vi "TimeInterpRotation_GetSample.vi"(9 "TimeStamp":dbl, 11 "TimeInterpRotation":T1 {"RotationValues"."SIN" format="%13.4f"; "RotationValues"."COS" format="%13.4f"; "RotationValues"."VALUE" format="%13.4f"}) -> (3 "OutputRotation":T2={"VALUE"=0.0, "COS"=1.0, "SIN"=0.0} {"SIN" format="%13.4f"; "COS" format="%13.4f"; "VALUE" format="%13.4f"})   [LabVIEW 2019, in "Trajectory_Library.lvlib"]
doc: "Calculate the output Y value for the provided X. This is done by interpolating through an array of X and Y pairs. The pairs must be ordered in increasing X value.\n\nInputs:\n - Function_Generator -- function generator data structure\n - Input Value -- The input value. \n\nOutputs:\n - Output Value -- Output value calcuated from the input value."
uses:
  Trajectory_Library.lvlib
  <vilib>/gmath/NI_Gmath.lvlib
  ROTATION2D.ctl
  TIME_INTERPOLATABLE_ROTATION.ctl
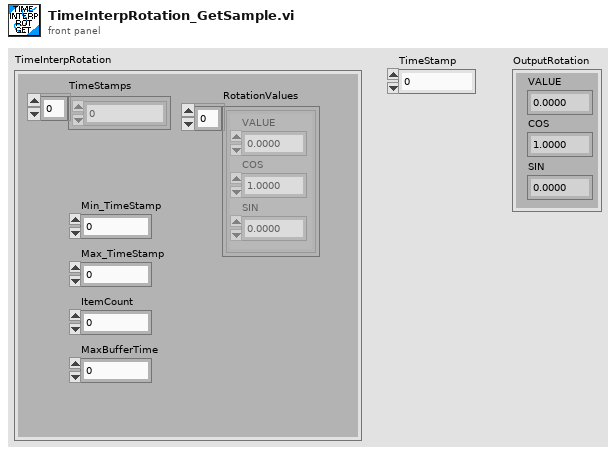
[diagram p1: front panel]
types:
  T1 = typedef "Trajectory_Library.lvlib/TIME_INTERPOLATABLE_ROTATION.ctl" = cluster{"TimeStamps":dbl[], "RotationValues":T2[], "Min_TimeStamp":dbl, "Max_TimeStamp":dbl, "ItemCount":i32, "MaxBufferTime":dbl}
  T2 = typedef "Trajectory_Library.lvlib/ROTATION2D.ctl" = cluster{"VALUE":dbl, "COS":dbl, "SIN":dbl}
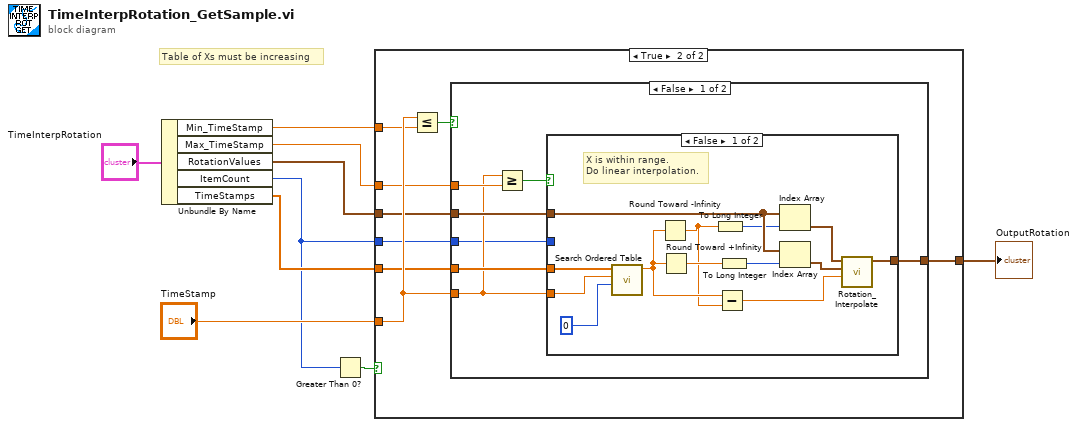
[diagram p0: block diagram]
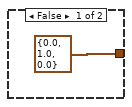
[diagram p2: hidden frame]
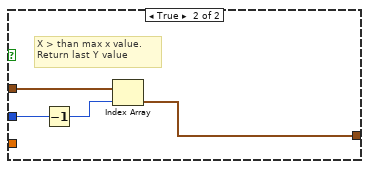
[diagram p3: hidden frame]
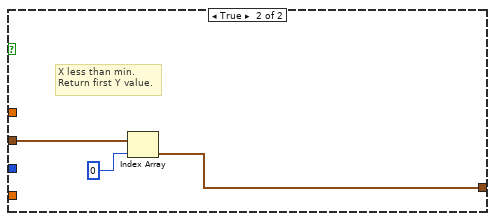
[diagram p4: hidden frame]
diagram:
  # "Table of Xs must be increasing"
  n1 = Unbundle By Name("TimeInterpRotation") -> ("Min_TimeStamp"=w6:dbl, "Max_TimeStamp"=w5:dbl, "RotationValues"=w3:T2[], "ItemCount"=w1:i32, "TimeStamps"=w4:dbl[])
  n2 = Greater Than 0?(x=w1) -> (x > 0?=w2:bool)
  n3 = case shown="True" w2 {
    tunnel: "TimeStamp" -> [_ w17]
    tunnel: [T2 {"VALUE"=0.0, "COS"=1.0, "SIN"=0.0} ("Table Y") w16] -> w8
    tunnel: w6 -> [_ w15]
    tunnel: w5 -> [_ w14]
    tunnel: w1 -> [_ w13]
    tunnel: w4 -> [_ w12]
    tunnel: w3 -> [_ w11]
    frame False {
    }
    frame True {
      n4 = Less Or Equal?(x=w17, y=w15) -> (x <= y?=w18:bool)
      n5 = case shown="False" w18 {
        tunnel: w11 -> [w23 w45]
        tunnel: [w22 w43] -> w16
        tunnel: w17 -> [w20 _]
        tunnel: w14 -> [w25 _]
        tunnel: w12 -> [w21 _]
        tunnel: w13 -> [w19 _]
        frame False {
          n6 = Greater Or Equal?(x=w20, y=w25) -> (x >= y?=w24:bool)
          n7 = case shown="False" w24 {
            tunnel: w23 -> [w34 w42]
            tunnel: [w35 w41] -> w22
            tunnel: w21 -> [w37 _]
            tunnel: w20 -> [w36 _]
            tunnel: w19 -> [_ w40]
            frame False {
              # "X is within range.  \nDo linear interpolation."
              n8 = call <vilib>:"Search Ordered Table.vi"("starting index"=0, "x value"=w36, "ordered x array"=w37) -> ("fractional index"=w28:dbl)  [unwired: 8 in]
              n9 = Round Toward -Infinity(1:w28) -> (0:w27:dbl)
              n10 = Round Toward +Infinity(x=w28) -> (ceil(x): smallest int >= x=w29:dbl)
              n11 = To Long Integer(number=w27) -> (32bit integer=w31:i32)
              n12 = Subtract(x=w28, y=w27) -> (x-y=w26:dbl)
              n13 = To Long Integer(number=w29) -> (32bit integer=w30:i32)
              n14 = Index Array(array=w34, index=w31) -> (element=w33:T2)
              n15 = Index Array(array=w34, index=w30) -> (element=w32:T2)
              n16 = call "Rotation_Interpolate.vi"("T"=w26, "EncValue ROTATION"=w32, "in ROTATION"=w33) -> ("Interpolated ROTATION"=w35:T2)  [unwired: 8 in]
            }
            frame True {
              # "X > than max x value.   \nReturn last Y value"
              n17 = Decrement(x=w40) -> (x-1=w39:i32)
              n18 = Index Array(array=w42, index=w39) -> (element=w41:T2)
            }
          }
        }
        frame True {
          # "X less than min.   \nReturn first Y value."
          n19 = Index Array(array=w45, index=0) -> (element=w43:T2)
        }
      }
    }
  }
  "OutputRotation" <- w8
